vi "Read_TDMS.vi"() -> ()   [LabVIEW 2018]
panel:
  out "웨이브폼 그래프":waveform(dbl)[](graph)
  out "데이터":waveform(dbl)[](array[waveform])
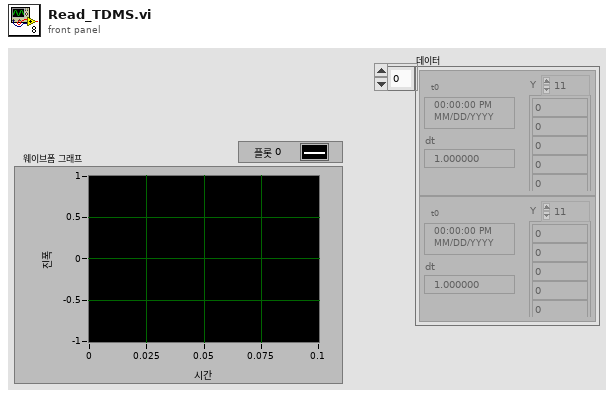
[diagram p1: front panel]
types:
  T1 = enum16{"open", "open or create", "create or replace", "create", "open (read-only)"}
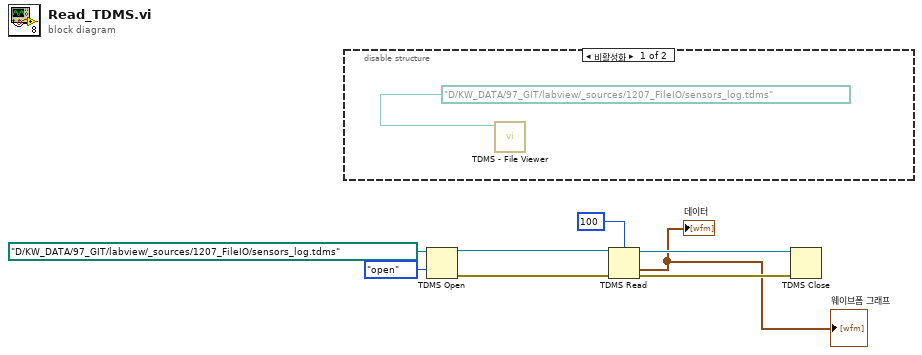
[diagram p0: block diagram]
diagram:
  n1 = disable-structure shown="비활성화" {
    frame Disabled {
      n2 = call <vilib>:"TDMS - File Viewer.vi"("file path"=path "D:/KW_DATA/97_GIT/labview/_sources/1207_FileIO/sensors_log.tdms") -> ()  [unwired: 5 in, 2 out]
    }
    frame Enabled {
    }
  }
  n3 = TDMS Open(10:T1."open" ("동작(0:open)"), 11:path "D:/KW_DATA/97_GIT/labview/_sources/1207_FileIO/sensors_log.tdms" ("파일 경로")) -> (0:w7:errorcluster, 3:w8:refnum<k34>)  [unwired: 5 in]
  n4 = TDMS Read(0:w8, 2:i64 100 ("카운트(-1: 전체)"), 11:w7) -> (4:w6:refnum<k34>, 10:→"데이터" →"웨이브폼 그래프":waveform(dbl)[], 15:w5:errorcluster)  [unwired: 5 in, 3 out]
  n5 = TDMS Close(8:w5, 11:w6) -> ()  [unwired: 2 out]
